vi "Listener Ref.vi"(6 "Action":T1, 8 "Error In":errorcluster, 11 "Listener Ref":refnum<k24>) -> (0 "Error Out":errorcluster, 3 "Listener Ref":refnum<k24>)   [LabVIEW 2014, in "SSL Lib.lvlib"]
doc: "VI Function: This is a Functional global that stores the TCP listener reference.\n\nVI Version: 1.0\n\nVI Author: Runjhun Agarwal"
uses:
  <userlib>/SSL Library/SSL Lib.lvlib
  <userlib>/SSL Library/Controls/Ref.ctl
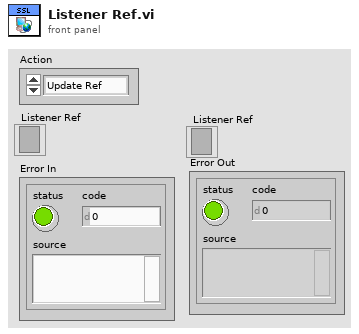
[diagram p1: front panel]
types:
  T1 = typedef "Ref.ctl" = enum16{"Update Ref", "Read Ref", "Close Ref"}
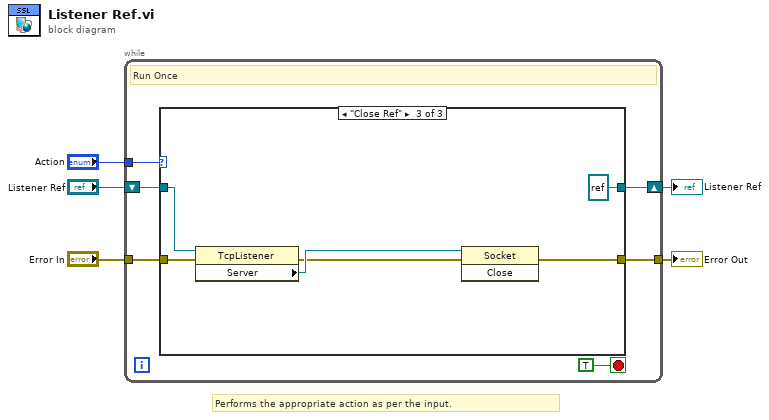
[diagram p0: block diagram]
diagram:
  # "Performs the appropriate action as per the input."
  n1 = while {
    tunnel: "Action" -> [w10]
    shift-right: [w8] -> w3
    shift-left: "Listener Ref" -> [w9]
    tunnel: "Error In" -> [w7]
    tunnel: [w6] -> w2
    stop <- TRUE stop-if-true
    # "Run Once"
    n2 = case shown="\"Close Ref\"" w10 {
      tunnel: w9 -> [w12 w15 w20]
      tunnel: [w12 w15 refnum<k24> refnum ("Listener Ref")] -> w8
      tunnel: w7 -> [w13 w14 w19]
      tunnel: [w13 w14 w18] -> w6
      frame "Update Ref" {
      }
      frame "Read Ref", Default {
      }
      frame "Close Ref" {
        n3 = property class="TcpListener"(reference=w20, error in=w19) -> (error out=w16:errorcluster, "Server"=w17:refnum<k24>)  [unwired: 1 out]
        n4 = invoke class="Socket" method="Close"(reference=w17, error in=w16) -> (error out=w18:errorcluster)  [unwired: 1 in, 2 out]
      }
    }
  }
  "Listener Ref" <- w3
  "Error Out" <- w2
